vi "Read inserts profiles.vi"(6 "error in (no error)":errorcluster, 8 "File Name":string="Target inserts profiles", 9 "Insert name":enum16{"Insert #1", "Insert #2", "Calib insert"}(ring)) -> (0 "error out":errorcluster, 3 "top cup length":dbl)   [LabVIEW 2019]
uses:
  <vilib>/Utility/config.llb/Read Key (Double).vi
  <vilib>/Utility/config.llb/NI_LVConfig.lvlib
panel:
  out "appended path":path
  out "concatenated string":string
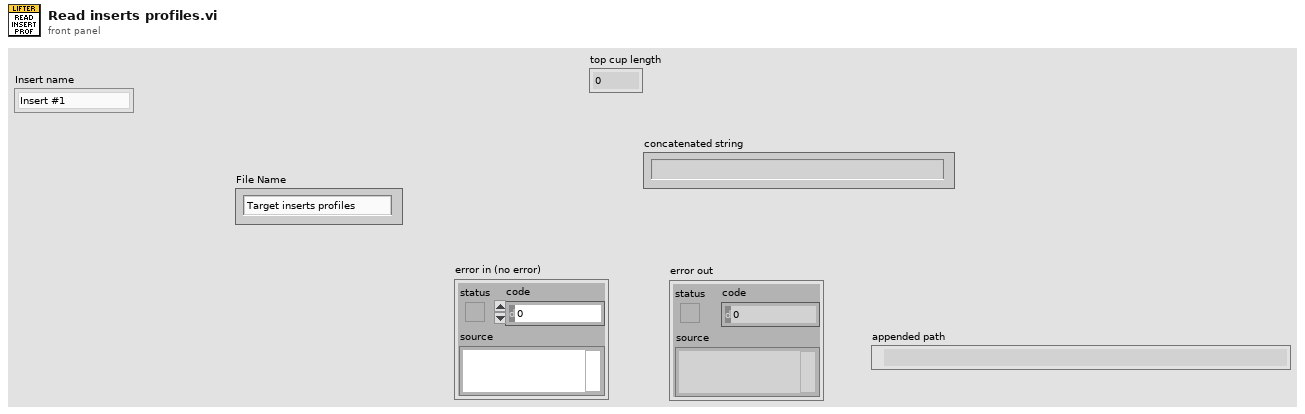
[diagram p1: front panel]
types:
  T1 = typedef "NI_LVConfig.lvlib/Config Data RefNum.ctl" = refnum<k1>
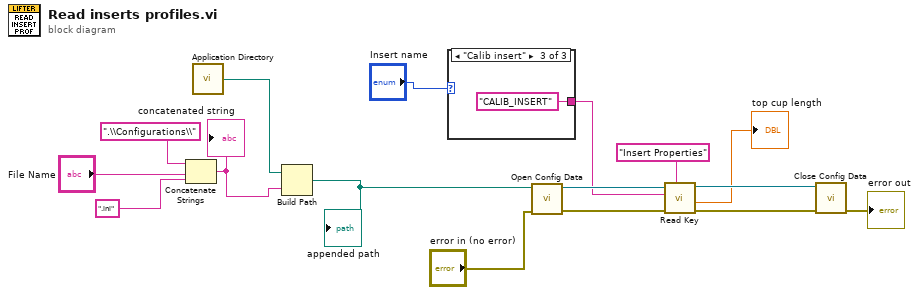
[diagram p0: block diagram]
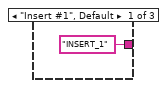
[diagram p2: hidden frame]
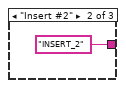
[diagram p3: hidden frame]
diagram:
  n1 = Concatenate Strings(".\\Configurations\\" ("string"), "File Name", ".ini" ("string")) -> (w14:string)
  "concatenated string" <- w14
  n2 = call <vilib>:"Application Directory.vi"() -> ("Application Directory"=w12:path)
  n3 = Build Path(base path=w12, name or relative path=w14) -> (appended path=w9:path)
  "appended path" <- w9
  n4 = case shown="\"Calib insert\"" "Insert name" {
    tunnel: ["INSERT_1" ("section") "INSERT_2" ("section") "CALIB_INSERT" ("section")] -> w5
    frame "Insert #1", Default {
    }
    frame "Insert #2" {
    }
    frame "Calib insert" {
    }
  }
  n5 = call <vilib>:"Open Config Data.vi"("error in (no error)"="error in (no error)", "configuration file path"=w9) -> ("error out"=w3:errorcluster, "refnum"=w7:T1)  [unwired: 7 in, 1 out]
  n6 = call-poly <vilib>:"Read Key.vi"("section"="Insert Properties", "error in (no error)"=w3, "key"=w5, "refnum"=w7) -> ("error out"=w4:errorcluster, "value"=→"top cup length":dbl, "refnum out"=w6:T1)  [unwired: 4 in, 1 out]
  n7 = call <vilib>:"Close Config Data.vi"("error in (no error)"=w4, "refnum"=w6) -> ("error out"=→"error out":errorcluster)  [unwired: 8 in, 1 out]
